vi "ISOLATION FGV.vi"(7 "STATES":T1=enum."CLOSE", 8 "error in (no error)":errorcluster) -> (0 "error out":errorcluster)   [LabVIEW 2018]
uses:
  CONTROLS/STATES ISOLATION.ctl
  <vilib>/xnet/xnet.llb/XNET Create Session (Signal Output Single-point).vi
  <vilib>/xnet/xnet.llb/XNET Write (Signal Single-point).vi
panel:
  out "session out 2":refnum<k21>
  in  "CAN SIGNAL":string
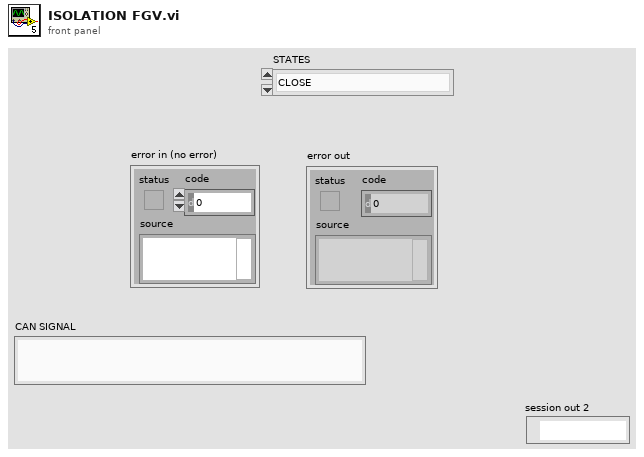
[diagram p1: front panel]
types:
  T1 = typedef "STATES ISOLATION.ctl" = enum16{"OPEN", "WRITE CAN", "CLOSE"}
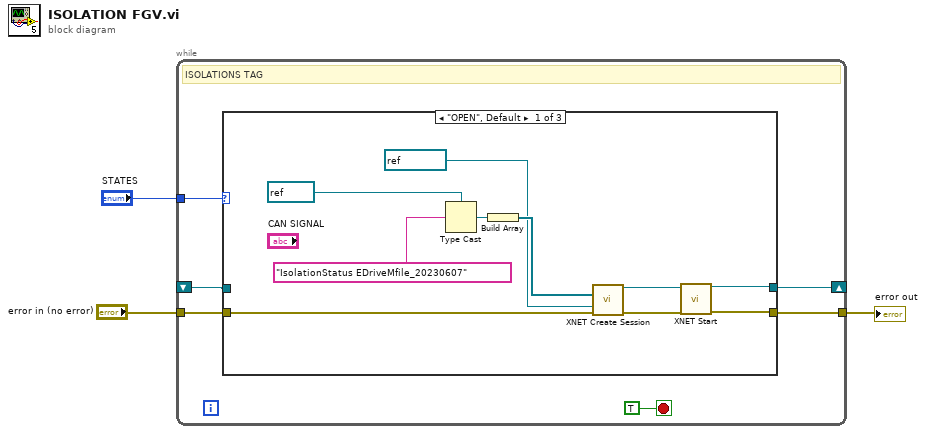
[diagram p0: block diagram]
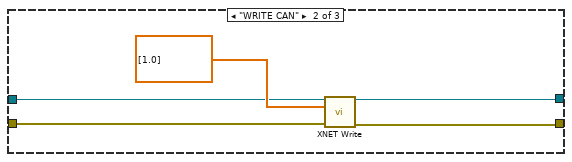
[diagram p2: hidden frame]
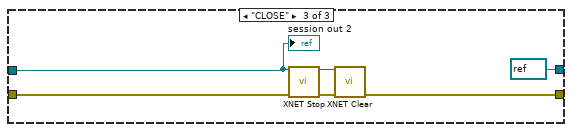
[diagram p3: hidden frame]
diagram:
  n1 = while {
    tunnel: "STATES" -> [w8]
    shift-right: [w7] -> _
    shift-left: _ -> [w4]
    tunnel: [w6] -> w1
    tunnel: "error in (no error)" -> [w5]
    stop <- TRUE stop-if-true
    # "ISOLATIONS TAG"
    n2 = case shown="\"OPEN\", Default" w8 {
      tunnel: [w11 w22 refnum<k21> refnum ("session out")] -> w7
      tunnel: [w12 w23 w27] -> w6
      tunnel: w5 -> [w15 w20 w28]
      tunnel: w4 -> [_ w21 w25]
      frame "OPEN", Default {
        n3 = Type Cast(type=refnum<k21> " " ("XNET Signal"), x="IsolationStatus EDriveMfile_20230607") -> (*(type *) &x=w18:refnum<k21>)
        n4 = Build Array(w18) -> (w19:refnum<k21>[])
        n5 = call-poly <vilib>:"XNET Create Session.vi"("signal list"=w19, "interface"=refnum<k21> "CAN1" ("Select Interface"), "error in (no error)"=w15) -> ("session out"=w14:refnum<k21>, "error out"=w13:errorcluster)  [unwired: 11 out]
        n6 = call <vilib>:"XNET Start.vi"("session in"=w14, "error in (no error)"=w13) -> ("session out"=w11:refnum<k21>, "error out"=w12:errorcluster)  [unwired: 12 in]
      }
      frame "WRITE CAN" {
        n7 = call-poly <vilib>:"XNET Write.vi"("session in"=w21, "data"=dbl[] [1.0], "error in (no error)"=w20) -> ("session out"=w22:refnum<k21>, "error out"=w23:errorcluster)  [unwired: 11 in]
      }
      frame "CLOSE" {
        n8 = call <vilib>:"XNET Stop.vi"("session in"=w25, "error in (no error)"=w28) -> ("session out"=w29:refnum<k21>, "error out"=w30:errorcluster)  [unwired: 12 in]
        n9 = call <vilib>:"XNET Clear.vi"("session in"=w29, "error in (no error)"=w30) -> ("error out"=w27:errorcluster)  [unwired: 13 in]
        "session out 2" <- w25
      }
    }
  }
  "error out" <- w1
